vi "SendEncryptedEndpointAuth.vi"(8 "error in (no error)":errorcluster, 10 "Update Password":T10, 11 "config":T1) -> (0 "error out":errorcluster)   [LabVIEW 2017, in "ServerComm.lvlib"]
uses:
  <vilib>/addons/InsightCM/Devices/Shared/Common/ServerComm/ServerComm.lvlib
  <vilib>/addons/InsightCM/Devices/Shared/Common/ServerComm/controls/UpdatePassword.ctl
  <vilib>/addons/InsightCM/Devices/Shared/Common/ServerComm/controls/config.ctl
  <vilib>/addons/InsightCM/MessageBus/TcpApi/controls/TcpMessageReference.ctl
  <vilib>/addons/InsightCM/MessageBus/Base/controls/ConnectionInfo.ctl
  <vilib>/addons/InsightCM/SRP/controls/DVR_data.ctl
  <vilib>/addons/InsightCM/SRP/controls/data.ctl
  <vilib>/addons/InsightCM/Devices/Shared/Common/ServerComm/controls/ConnectedStatusDvr.ctl
  <vilib>/addons/InsightCM/Devices/Shared/Common/ServerComm/controls/ConnectionStatus.ctl
  <vilib>/addons/InsightCM/Devices/Shared/Common/ServerComm/controls/DataSendStatus.ctl
  <vilib>/addons/InsightCM/Devices/Shared/Common/ServerComm/controls/DataSendMode.ctl
  <vilib>/addons/InsightCM/Devices/Shared/Common/ServerComm/controls/ReconnectData.ctl
  <vilib>/addons/InsightCM/Devices/Shared/Common/ServerComm/controls/ProvisioningVersionInfo.ctl
  <vilib>/addons/InsightCM/MessageBus/MessageLibrary/Provisioning/controls/ProvisioningSetEndpointAuthsRoutedMessageBody.ctl
  <vilib>/addons/InsightCM/MessageBus/Base/controls/WirelessEndpointAuth.ctl
  <vilib>/addons/InsightCM/SRP/SRP.lvlib
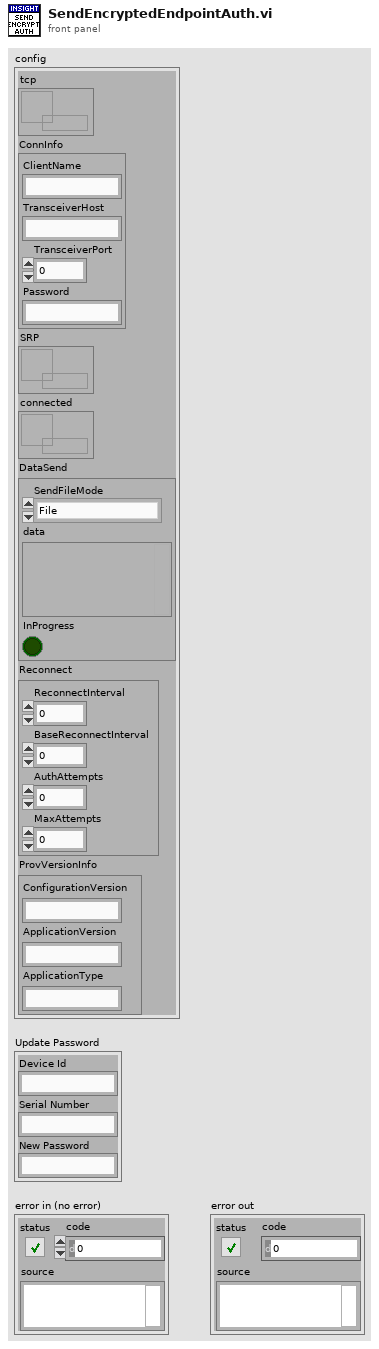
[diagram p1: front panel]
types:
  T1 = typedef "ServerComm.lvlib/config.ctl" = cluster{"tcp":T2, "ConnInfo":T3, "SRP":T4, "connected":T5, "DataSend":T6, "Reconnect":T8, "ProvVersionInfo":T9}
  T2 = typedef "TcpMessageReference.ctl" = refnum<data-value>
  T3 = typedef "ConnectionInfo.ctl" = cluster{"ClientName":string, "TransceiverHost":string, "TransceiverPort":u16, "Password":string}
  T4 = typedef "SRP.lvlib/DVR_data.ctl" = refnum<data-value>
  T5 = typedef "ServerComm.lvlib/ConnectedStatusDvr.ctl" = refnum<data-value>
  T6 = typedef "ServerComm.lvlib/DataSendStatus.ctl" = cluster{"SendFileMode":T7, "data":variant, "InProgress":bool}
  T7 = typedef "ServerComm.lvlib/DataSendMode.ctl" = enum16{"File", "InMemoryFile", "Stream", "StreamFileBlock", "ByteArray", "NoOp", "UnknownData"}
  T8 = typedef "ServerComm.lvlib/ReconnectData.ctl" = cluster{"ReconnectInterval":dbl, "BaseReconnectInterval":dbl, "AuthAttempts":i32, "MaxAttempts":i32}
  T9 = typedef "ServerComm.lvlib/ProvisioningVersionInfo.ctl" = cluster{"ConfigurationVersion":string, "ApplicationVersion":string, "ApplicationType":string}
  T10 = typedef "ServerComm.lvlib/UpdatePassword.ctl" = cluster{"Device Id":string, "Serial Number":string, "New Password":string}
  T11 = typedef "WirelessEndpointAuth.ctl" = cluster{"SerialNumber":string, "Password":string, "Reset":bool}
  T12 = typedef "ProvisioningSetEndpointAuthsRoutedMessageBody.ctl" = cluster{"DeviceId":string, "IV":u8[], "AuthList":u8[]}
  T13 = typedef "Message.ctl" = cluster{"Header":T14, "Body":u8[]}
  T14 = typedef "MessageHeader.ctl" = cluster{"MessageName":string, "Timestamp":i64, "CorrelationId":string, "ContentType":string, "RoutingKey":string, "Properties":T15[]}
  T15 = typedef "KeyValuePair.ctl" = cluster{"Key":string, "Value":string}
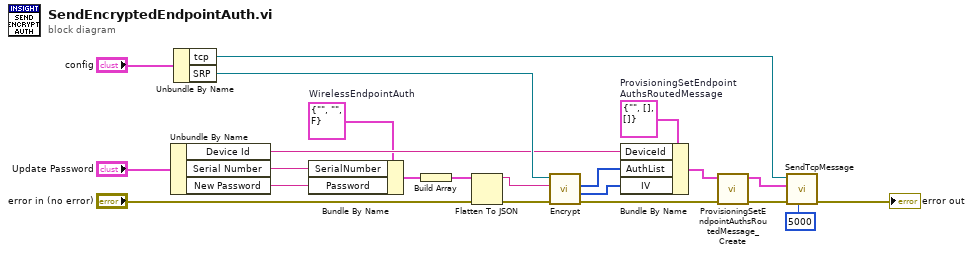
[diagram p0: block diagram]
diagram:
  w9 = T11 {"SerialNumber"="", "Password"="", "Reset"=FALSE}  # WirelessEndpointAuth
  w18 = T12 {"DeviceId"="", "IV"=[], "AuthList"=[]}  # ProvisioningSetEndpointAuthsRoutedMessage
  n1 = Unbundle By Name("Update Password") -> ("Device Id"=w10:string, "Serial Number"=w8:string, "New Password"=w7:string)
  n2 = Unbundle By Name("config") -> ("tcp"=w16:T2, "SRP"=w15:T4)
  n3 = Bundle By Name(cluster=w9, "SerialNumber"=w8, "Password"=w7) -> (w6:T11)
  n4 = Build Array(w6) -> (w3:T11[])
  n5 = Flatten To JSON(anything=w3, error in (no error)="error in (no error)") -> (JSON string=w2:string, 11:w4:errorcluster)  [unwired: 1 in]
  n6 = call <vilib>:"Encrypt.vi"("error in (no error)"=w4, "input"=w2, "srp"=w15) -> ("error out"=w14:errorcluster, "IV"=w13:u8[], "output"=w12:u8[])  [unwired: 5 in, 1 out]
  n7 = Bundle By Name(cluster=w18, "DeviceId"=w10, "AuthList"=w12, "IV"=w13) -> (w17:T12)
  n8 = call <vilib>:"ProvisioningSetEndpointAuthsRoutedMessage_Create.vi"("error in (no error)"=w14, "ProvisioningSetEndpointAuthsRoutedMessage"=w17) -> ("error out"=w19:errorcluster, "Message"=w20:T13)  [unwired: 8 in]
  n9 = call <vilib>:"SendTcpMessage.vi"("timeout (5 sec)"=5000, "error in (no error)"=w19, "message"=w20, "connection ID in"=w16) -> ("error out"=→"error out":errorcluster)  [unwired: 5 in, 2 out]
